vi "JSON To Variant.vi"(8 "error in (no error)":errorcluster, 9 "datatype and defaults":variant, 11 "JSON Value in":refnum<class "JSON Value.lvclass">) -> (0 "error out":errorcluster, 1 "defaulted keys":string[](array[string]), 2 "Variant":variant)   [LabVIEW 2016, in "JSFL Variant Support.lvlib"]
doc: "Populates a variant with the data contained in the given JSON instance. Valid types for datatype and defaults are: string, boolean, double, and a cluster of named controls of strings, booleans, doubles, or nested clusters.\n\nIf a given cluster contains values that aren't present in the JSON Object instance, the value in the datatype and defaults control is used instead and the defaulted keys output will contain the name of the path in the cluster to the control."
uses:
  JSFL Variant Support.lvlib
  JSON Value.lvclass
  Read Value/Read value (Numeric).vi
  Read Value/Read value (Boolean).vi
  Read Value/Read value (String).vi
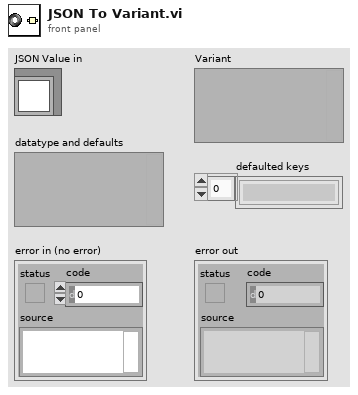
[diagram p1: front panel]
types:
  T1 = typedef "JSON Value.lvclass/JSON Types.ctl" = enum16{"String", "Numeric", "Boolean", "NULL", "Object", "Array"}
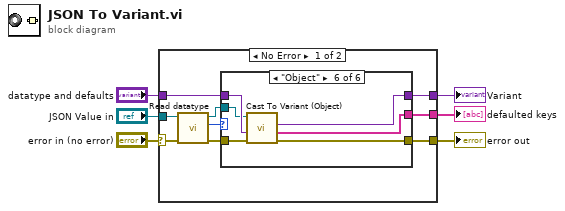
[diagram p0: block diagram]
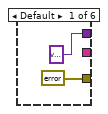
[diagram p2: hidden frame]
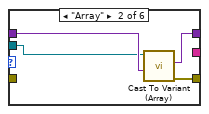
[diagram p3: hidden frame]
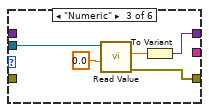
[diagram p4: hidden frame]
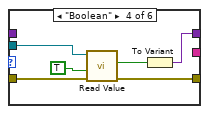
[diagram p5: hidden frame]
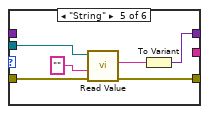
[diagram p6: hidden frame]
diagram:
  n1 = case shown="No Error" "error in (no error)" {
    selector: "error in (no error)" -> [w8 w46]
    tunnel: [w13 w46] -> w5
    tunnel: "JSON Value in" -> [w11 _]
    tunnel: "datatype and defaults" -> [w14 w45]
    tunnel: [w15 w45] -> w2
    tunnel: [w12 _] -> w1
    frame No Error {
      n2 = call "Read datatype.vi"("error in (no error)"=w8, "JSON Value in"=w11) -> ("error out"=w7:errorcluster, "datatype"=w9:T1, "JSON Value out"=w10:refnum<class "JSON Value.lvclass">)  [unwired: 7 in]
      n3 = case shown="\"Object\"" w9 {
        tunnel: w10 -> [_ w18 w24 w30 w36 w39]
        tunnel: [variant ("datatype and defaults") w19 w25 w32 w37 w43] -> w15
        tunnel: w14 -> [_ w20 _ _ _ w44]
        tunnel: w7 -> [_ _ _ w27 w33 w40]
        tunnel: [errorcluster {"status"=TRUE, "code"=-1000, "source"="Default not implemented. Please specify expected type"} ("error out") w21 w26 w31 w38 w42] -> w13
        tunnel: [_ _ _ _ _ w41] -> w12
        frame Default {
        }
        frame "Array" {
          n4 = call "Cast To Variant (Array).vi"("datatype and defaults"=w20, "JSON Value in"=w18) -> ("error out"=w21:errorcluster, "Variant"=w19:variant)  [unwired: 8 in]
        }
        frame "Numeric" {
          n5 = call-poly "Read Value.vi"("default value"=0.0, "JSON Numeric in"=w24) -> ("error out"=w26:errorcluster, "value"=w23:dbl)  [unwired: 8 in]
          n6 = To Variant(anything=w23) -> (Variant=w25:variant)
        }
        frame "Boolean" {
          n7 = call-poly "Read Value.vi"("error in (no error)"=w27, "default value"=TRUE, "JSON Boolean in"=w30) -> ("error out"=w31:errorcluster, "value"=w29:bool)  [unwired: 7 in]
          n8 = To Variant(anything=w29) -> (Variant=w32:variant)
        }
        frame "String" {
          n9 = call-poly "Read Value.vi"("error in (no error)"=w33, "default value"="", "JSON String in"=w36) -> ("error out"=w38:errorcluster, "value"=w35:string)  [unwired: 7 in]
          n10 = To Variant(anything=w35) -> (Variant=w37:variant)
        }
        frame "Object" {
          n11 = call "Cast To Variant (Object).vi"("error in (no error)"=w40, "datatype and defaults"=w44, "JSON Value in"=w39) -> ("error out"=w42:errorcluster, "defaulted keys"=w41:string[], "Variant"=w43:variant)  [unwired: 6 in]
        }
      }
    }
    frame Error {
    }
  }
  "error out" <- w5
  "Variant" <- w2
  "defaulted keys" <- w1
